vi "ToString.vi"(8 "error in (no error)":errorcluster, 11 "Collection Distinct in":refnum<class "Collection Distinct.lvclass">) -> (0 "error out":errorcluster, 2 "String":string, 3 "Collection Distinct out":refnum<class "Collection Distinct.lvclass">)   [LabVIEW 2017, in "Transparent Assertions.lvlib" / "Constraints.lvlib" / "Collection Distinct.lvclass"]
doc: "Returns a string representation of the object."
uses:
  Collection Distinct.lvclass
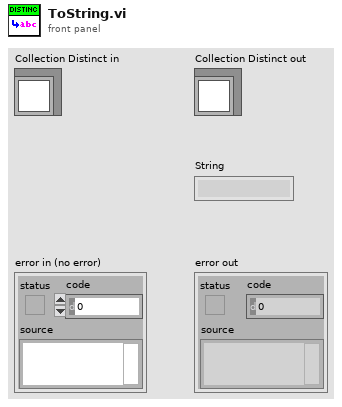
[diagram p1: front panel]
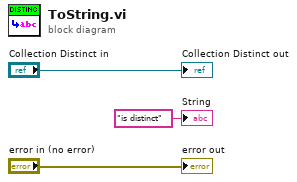
[diagram p0: block diagram]
diagram:
  "error out" <- "error in (no error)"
  "Collection Distinct out" <- "Collection Distinct in"
  "String" <- "is distinct" ("String")
